vi "Read Joystick Axis.vi"(11 "Joystick 0":dbl[](array[numeric])) -> ()   [LabVIEW 2020]
uses:
  Robot Global Data.vi
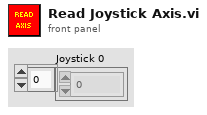
[diagram p1: front panel]
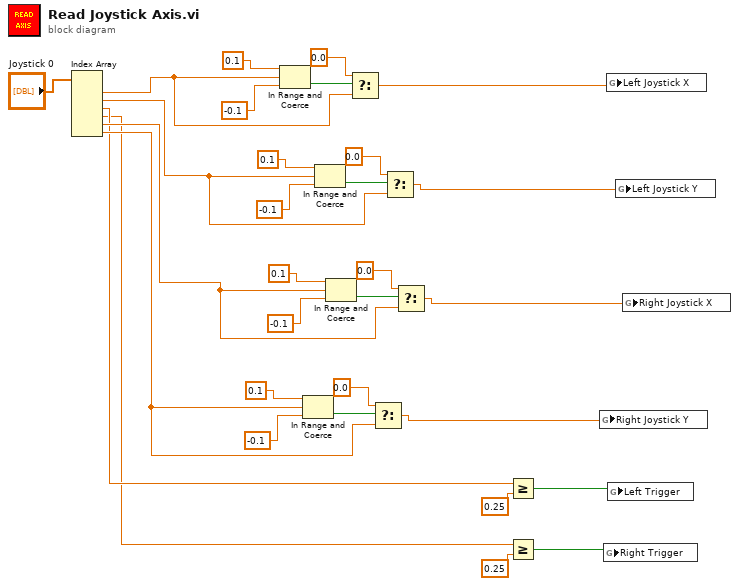
[diagram p0: block diagram]
diagram:
  n1 = Index Array(array="Joystick 0") -> (element #1=w26:dbl, element #2=w21:dbl, element #3=w4:dbl, element #4=w1:dbl, element #5=w13:dbl, element #6=w7:dbl)  [unwired: 6 in]
  n2 = In Range and Coerce(upper limit=0.1, x=w26, lower limit=-0.1) -> (In Range?=w29:bool)  [unwired: 1 out]
  n3 = In Range and Coerce(upper limit=0.1, x=w7, lower limit=-0.1) -> (In Range?=w10:bool)  [unwired: 1 out]
  n4 = In Range and Coerce(upper limit=0.1, x=w21, lower limit=-0.1) -> (In Range?=w23:bool)  [unwired: 1 out]
  n5 = In Range and Coerce(upper limit=0.1, x=w13, lower limit=-0.1) -> (In Range?=w16:bool)  [unwired: 1 out]
  n6 = Select(t=0.0, s=w29, f=w26) -> (s? t:f=w27:dbl)
  n7 = Select(t=0.0, s=w10, f=w7) -> (s? t:f=w8:dbl)
  n8 = Select(t=0.0, s=w23, f=w21) -> (s? t:f=w20:dbl)
  n9 = Select(t=0.0, s=w16, f=w13) -> (s? t:f=w14:dbl)
  n10 = Greater Or Equal?(x=w4, y=0.25) -> (x >= y?=w6:bool)
  n11 = Greater Or Equal?(x=w1, y=0.25) -> (x >= y?=w2:bool)
  n12 = global write "Robot Global Data.vi" "Right Joystick Y"(w8) -> ()
  n13 = global write "Robot Global Data.vi" "Right Trigger"(w2) -> ()
  n14 = global write "Robot Global Data.vi" "Left Joystick X"(w27) -> ()
  n15 = global write "Robot Global Data.vi" "Left Trigger"(w6) -> ()
  n16 = global write "Robot Global Data.vi" "Left Joystick Y"(w20) -> ()
  n17 = global write "Robot Global Data.vi" "Right Joystick X"(w14) -> ()
